vi "Content-Type Map.vi"(7 "Add Content-Type":string, 10 "File Extension":string, 11 "Action (Lookup)":T1) -> (2 "Extension Not Found?":bool, 3 "Extension Content-Type":string)   [LabVIEW 2020, in "HTTP Utils.lvlib"]
uses:
  HTTP Utils.lvlib
  Content-Type DB Action.ctl
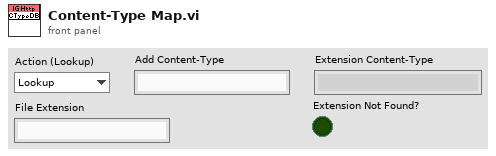
[diagram p1: front panel]
types:
  T1 = typedef "HTTP Utils.lvlib/Content-Type DB Action.ctl" = enum16{"Lookup", "Add"}
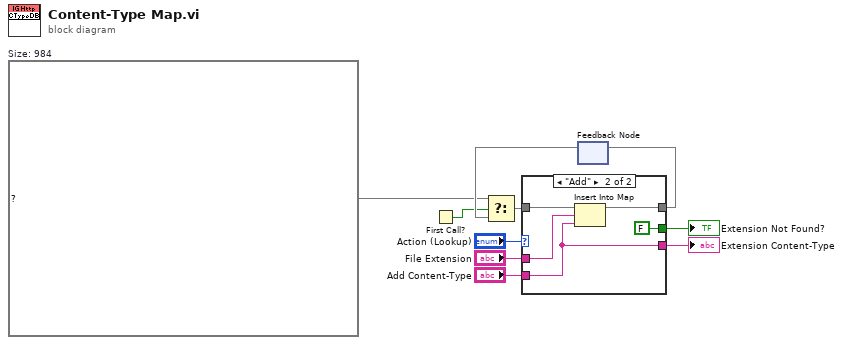
[diagram p0: block diagram]
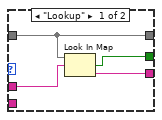
[diagram p2: hidden frame]
diagram:
  w2 = map{string, string} data[34436B]  # Size: 984
  n1 = First Call?() -> (First Call?: T/F=w1:bool)
  n2 = feedback #1() -> (w4:map{string, string})  [unwired: 1 in]
  n3 = Select(t=w2, s=w1, f=w4) -> (s? t:f=w3:map{string, string})
  n4 = case shown="\"Add\"" "Action (Lookup)" {
    tunnel: w3 -> [w14 w19]
    tunnel: [w14 w17] -> w9
    tunnel: "File Extension" -> [w13 w18]
    tunnel: "Add Content-Type" -> [_ w15]
    tunnel: [w12 w15] -> w6
    tunnel: [w11 FALSE ("key not found?")] -> w5
    frame "Lookup" {
      n5 = Look In Map(map=w14, key=w13) -> (key not found?=w11:bool, value=w12:string)  [unwired: 1 in]
    }
    frame "Add" {
      n6 = Insert Into Map(map in=w19, key=w18, value=w15) -> (map out=w17:map{string, string})  [unwired: 2 out]
    }
  }
  "Extension Content-Type" <- w6
  "Extension Not Found?" <- w5
  n7 = feedback-in #1(w9) -> ()
